vi "TestTCPServ.vi"() -> ()   [LabVIEW 2011]
uses:
  <vilib>/Platform/TimedLoop/XDataNode/timing_clust.ctl
  <vilib>/Platform/TimedLoop/XDataNode/nitl_modes.ctl
  <vilib>/Platform/TimedLoop/XDataNode/wakeup.ctl
  <vilib>/Platform/TimedLoop/XDataNode/XDataNode.xnode
  <vilib>/Platform/TimedLoop/XDataNode/XDNodeRunTimeDep.lvlib
panel:
  out "Error Out":errorcluster
  out "bytes written":i32
  in  "Boolean":bool
  out "NaN/Path/Refnum?":bool
  in  "port":i32=9000
  in  "String":string="localhost"
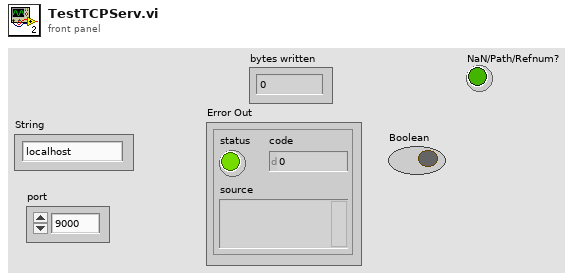
[diagram p1: front panel]
types:
  T1 = typedef "XDNodeRunTimeDep.lvlib/timing_clust.ctl" = cluster{"Expected End [f-1]":u64, "Actual End [f-1]":u64, "Finished Late? [f-1]":bool, "Expected End [i-1]":u64, "Actual End [i-1]":u64, "Finished Late? [i-1]":bool, "Expected Start [i]":u64, "Actual Start [i]":u64, "Expected Start [f]":u64, "Actual Start [f]":u64, "Source Name":string, "Structure Name":string, "Period":i64, "Deadline":i64, "Offset":i64, "Start":i64, "Priority":i32, "Timeout":i32, "Mode":T2, "Wakeup Reason":T3, "Error":errorcluster, "Source Type":string, "Secondary Source Type":string, "Global End Time":u64, "Global Start Time":u64, "Frame Duration":u64, "Iteration Duration":u64, "Assigned CPU":i32, "I/O Scan Engine Mode":u32}
  T2 = typedef "XDNodeRunTimeDep.lvlib/nitl_modes.ctl" = enum32{"No Change", "Process missed periods, maintain original phase", "Discard missed periods, maintain original phase", "Process missed periods, ignore original phase", "Discard missed periods, ignore original phase"}
  T3 = typedef "XDNodeRunTimeDep.lvlib/wakeup.ctl" = enum32{"Normal", "Aborted", "Asynchronous wakeup", "Timing source error", "Timed loop error", "Timeout"}
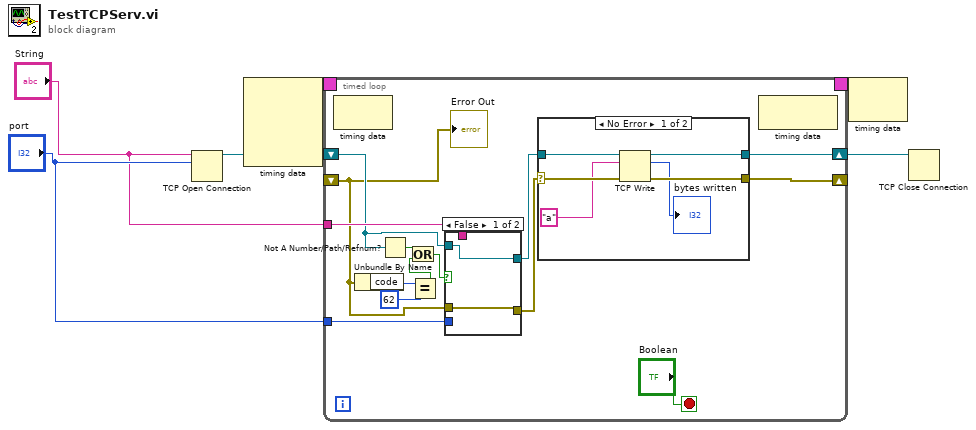
[diagram p0: block diagram]
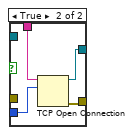
[diagram p2: hidden frame]
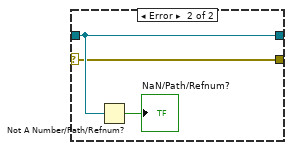
[diagram p3: hidden frame]
diagram:
  n1 = TCP Open Connection(address="String", remote port or service name="port") -> (connection ID=w6:refnum<k5>)  [unwired: 3 in, 1 out]
  n2 = node-c288() -> (w5:T1)  [unwired: 4 in]
  n3 = timed-loop {
    timing: w5 -> [_]
    timing-out: [_] -> w4
    shift-right: [w19] -> w3
    shift-left: w6 -> [w9]
    shift-right: [w18] -> _
    shift-left: _ -> [w7]
    tunnel: "port" -> [w12]
    tunnel: "String" -> [w11]
    stop <- "Boolean" stop-if-true
    n4 = node-c288() -> ()  [unwired: 1 in, 1 out]
    n5 = Unbundle By Name(w7) -> ("code"=w16:i32)
    n6 = Not A Number/Path/Refnum?(number/path/refnum=w9) -> (NaN/Path/Refnum?=w17:bool)
    n7 = Equal?(x=w16, y=62) -> (x = y?=w14:bool)
    n8 = Or(x=w17, y=w14) -> (x .or. y?=w13:bool)
    n9 = case shown="False" w13 {
      tunnel: w12 -> [_ w26]
      tunnel: w11 -> [_ w25]
      tunnel: [w22 w24] -> w10
      tunnel: w9 -> [w22 _]
      tunnel: [w21 w23] -> w8
      tunnel: w7 -> [w21 _]
      frame False {
      }
      frame True {
        n10 = TCP Open Connection(address=w25, remote port or service name=w26) -> (connection ID=w24:refnum<k5>, error out=w23:errorcluster)  [unwired: 3 in]
      }
    }
    n11 = case shown="No Error" w8 {
      selector: w8 -> [w29 w33]
      tunnel: w10 -> [w32 w35]
      tunnel: [w31 w35] -> w19
      tunnel: [w30 w33] -> w18
      frame No Error {
        n12 = TCP Write(connection ID=w32, data in="a", error in (no error)=w29) -> (connection ID out=w31:refnum<k5>, bytes written=→"bytes written":i32, error out=w30:errorcluster)  [unwired: 1 in]
      }
      frame Error {
        n13 = Not A Number/Path/Refnum?(number/path/refnum=w35) -> (NaN/Path/Refnum?=→"NaN/Path/Refnum?":bool)
      }
    }
    n14 = node-c288() -> ()  [unwired: 1 in, 1 out]
    "Error Out" <- w7
  }
  n15 = node-c288(w4) -> ()  [unwired: 1 out]
  n16 = TCP Close Connection(connection ID=w3) -> ()  [unwired: 2 in, 2 out]
